vi "Thread Parameters.Get ID.vi"(11 "Plugin in":refnum<class "Thread Parameters.lvclass">) -> (2 "id":i32, 3 "Plugin out":refnum<class "Thread Parameters.lvclass">)   [LabVIEW 2017, in "DSF Core.lvlib" / "Thread Parameters.lvclass"]
uses:
  Thread Parameters.lvclass
  Thread Parameters.lvclass/Thread Parameters.ctl
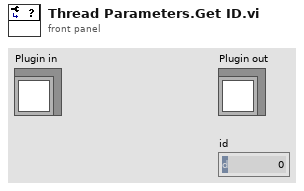
[diagram p1: front panel]
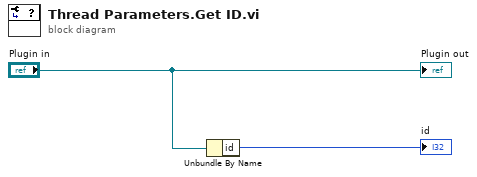
[diagram p0: block diagram]
diagram:
  n1 = Unbundle By Name("Plugin in") -> ("id"=→"id":i32)
  "Plugin out" <- "Plugin in"
